vi "Vision Research Phantom Series PhCon PhParamsChanged.vi"(0 "CN in":u32=1, 5 "Error In (no error)":errorcluster) -> (14 "CN out":u32=1, 16 "pChanged":bool, 19 "Error Out":errorcluster)   [LabVIEW 2013, in "VRI.lvlib"]
doc: "PhCon.dll\n\nPhParamsChanged\nHRESULT PhParamsChanged(UINT CN, PBOOL pChanged);\n\nParameters Description\nCN (in) Camera number.\npChanged (in) If TRUE, changes have been made to the camera's\n acqusition parameters.\nReturn HRESULT (0 = Ok)\nComments Use this function to determine whether another computer,\n remote control, or on-camera controls changed the \n acquisition parameters of the camera. If pChanged is\n TRUE, changes to the acquisition parameters have been\n made and a call to PhGetCineParams() should\n be made to read the new settings from the camera."
uses:
  VRI.lvlib
  Phantom DLLs/PhCon.dll
panel:
  # "For instructions on the use of this VI, press Ctrl+H to display the help window and move the mouse over the icon, controls, and indicators"
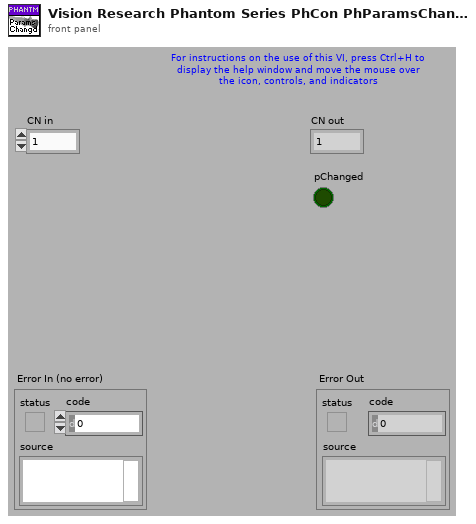
[diagram p1: front panel]
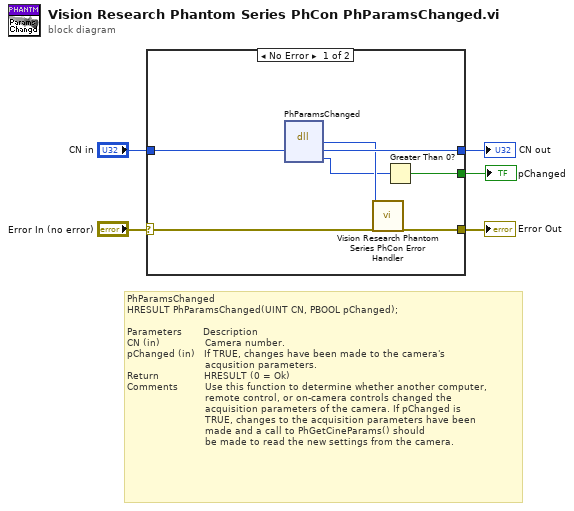
[diagram p0: block diagram]
diagram:
  # "PhParamsChanged\nHRESULT PhParamsChanged(UINT CN, PBOOL pChanged);\n\nParameters       Description\nCN (in)               Camera number.\npChanged (in)   If TRUE, changes have been made to the camera's\n                          acqusition parameters.\nReturn               HRESULT (0 = Ok)\nComments         Use this function to determine whether another computer,\n                          remote control, or on-camera controls changed the \n                          acquisition parameters of the camera. If pChanged is\n                          TRUE, changes to the acquisition parameters have been\n                          made and a call to PhGetCineParams() should\n                          be made to read the new settings from the camera."
  n1 = case shown="No Error" "Error In (no error)" {
    selector: "Error In (no error)" -> [w12 w14]
    tunnel: [w11 w14] -> w4
    tunnel: "CN in" -> [w10 w13]
    tunnel: [w9 w13] -> w2
    tunnel: [w8 _] -> w1
    frame No Error {
      n2 = dll-call lib="C:/Projects/SDK/32-bit/Vision Research Phantom Series Labview Driver/Phantom DLLs/PhCon.dll" fn="PhParamsChanged"("CN"=w10) -> ("HRESULT"=w7:i32, "CN"=w9:u32, "pChanged"=w6:i32)  [unwired: 3 in, 3 out]
      n3 = call "Vision Research Phantom Series PhCon Error Handler.vi"("ErrNo"=w7, "Error In (no error)"=w12) -> ("Error Out"=w11:errorcluster)  [unwired: 17 out]
      n4 = Greater Than 0?(x=w6) -> (x > 0?=w8:bool)
    }
    frame Error {
    }
  }
  "Error Out" <- w4
  "CN out" <- w2
  "pChanged" <- w1
